vi "GetImage.vi"(10 "FileName":string="andre", 11 "VISA resource name":refnum<visa-resource-name>) -> ()   [LabVIEW 2014]
panel:
  out "Receive Buffer_MP":u8[](array[numeric])
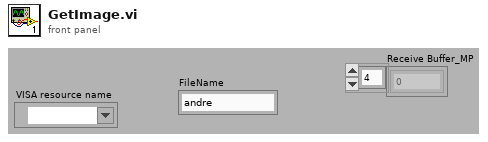
[diagram p1: front panel]
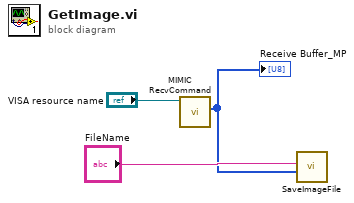
[diagram p0: block diagram]
diagram:
  n1 = call "MIMIC RecvCommand.vi"("VISA resource name"="VISA resource name") -> ("Receive Buffer_MP"=w2:u8[])  [unwired: 3 in, 3 out]
  "Receive Buffer_MP" <- w2
  n2 = call "SaveImageFile.vi"("ImagData"=w2, "FileName"="FileName") -> ()  [unwired: 7 in, 3 out]
